vi "main.vi"() -> ()   [LabVIEW 2012]
panel:
  out "update flag":dbl[](array[numeric])
  out "Current Chart":dbl(graph)
  out "Temperature Chart":dbl(graph)
  in  "stop":bool
  in  "Pulse Width":dbl
  in  "Interlock":bool
  in  "Override":bool
  out "Laser Current":dbl(slide) scale=800.0..1024.0
  out "Laser Temperature":dbl(slide) scale=10.0..50.0
  in  "COMPort":refnum<visa-resource-name>
  in  "Input Source":bool
  in  "Period":dbl
  in  "Delay":dbl
  # "Internal"
  # "External"
  # "Interlock"
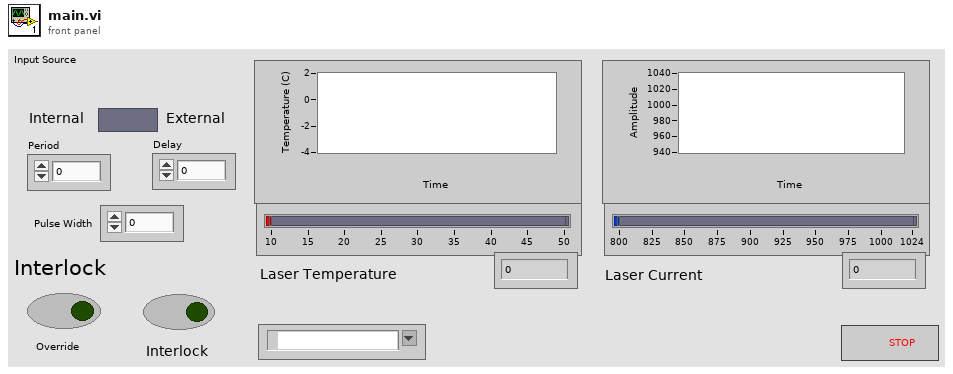
[diagram p1: front panel]
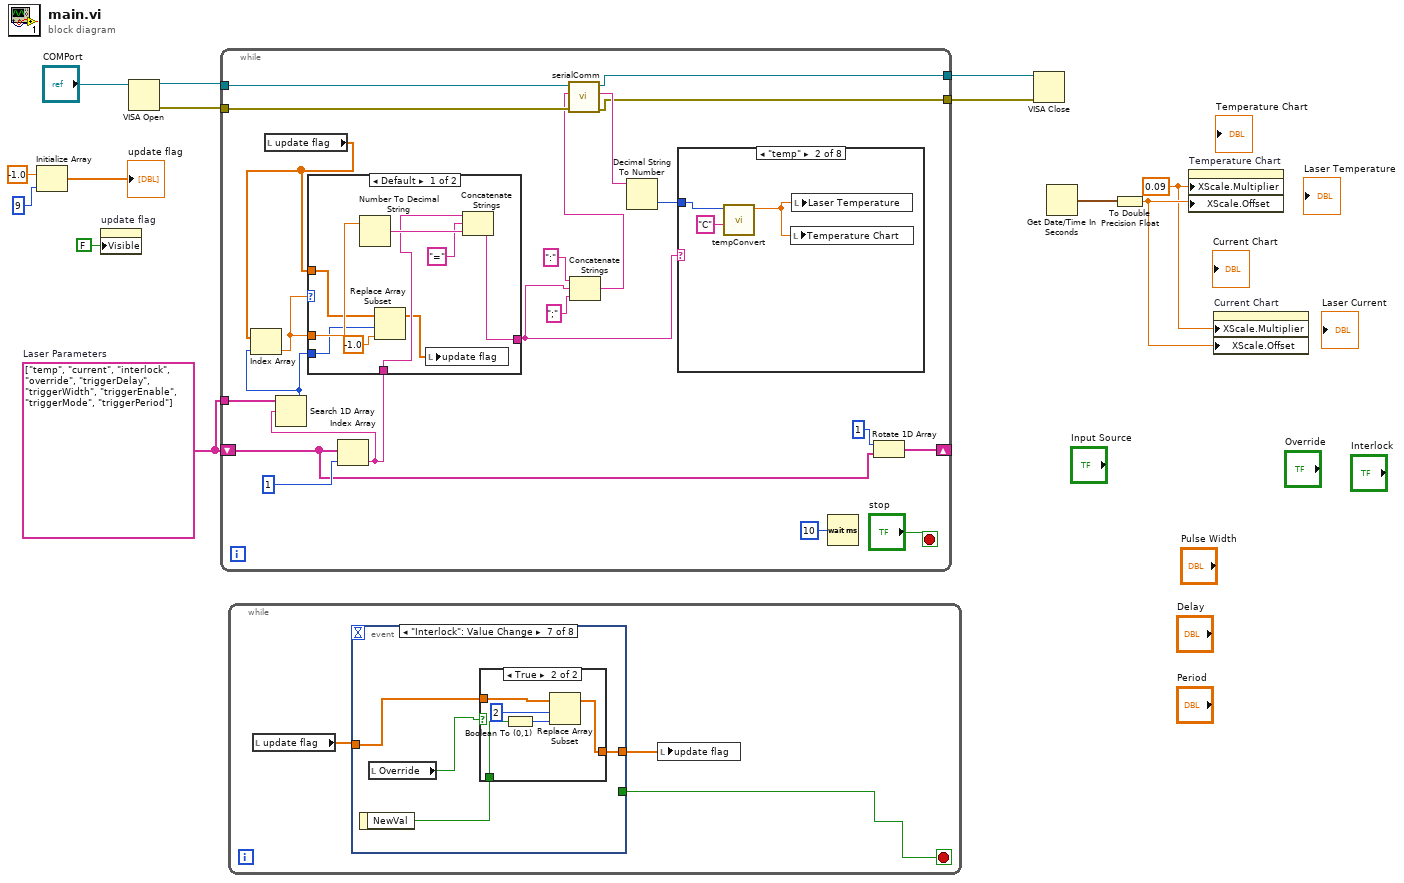
[diagram p0: block diagram]
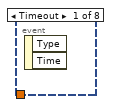
[diagram p2: hidden frame]
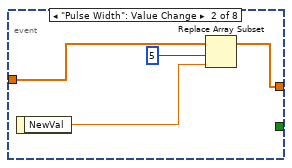
[diagram p3: hidden frame]
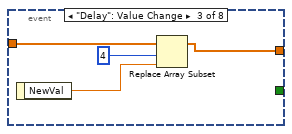
[diagram p4: hidden frame]
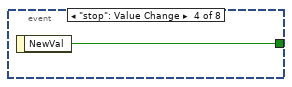
[diagram p5: hidden frame]
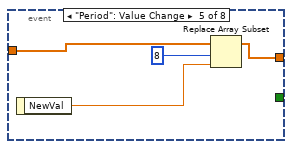
[diagram p6: hidden frame]
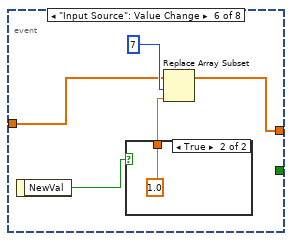
[diagram p7: hidden frame]
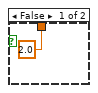
[diagram p8: hidden frame]
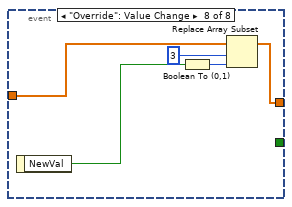
[diagram p10: hidden frame]
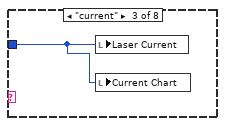
[diagram p13: hidden frame]
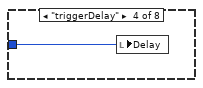
[diagram p14: hidden frame]
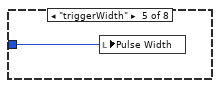
[diagram p15: hidden frame]
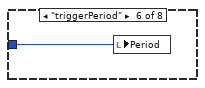
[diagram p16: hidden frame]
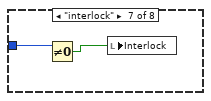
[diagram p17: hidden frame]
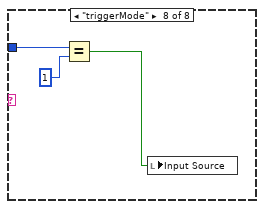
[diagram p18: hidden frame]
diagram:
  w6 = 0.09 ("X Scale.Offset and Multiplier:Multiplier")
  w5 = string[] ["temp", "current", "interlock", "override", "triggerDelay", "triggerWidth", "triggerEnable", "triggerMode", "triggerPeriod"]  # Laser Parameters
  n1 = Initialize Array(-1.0 ("element"), 9 ("dimension size")) -> (→"update flag":dbl[])
  n2 = property on="update flag" class="Arr (strict)"("Visible"=FALSE) -> ()  [unwired: 2 in, 2 out]
  n3 = VISA Open(VISA resource name="COMPort") -> (VISA resource name=w12:refnum<visa-resource-name>, error out=w11:errorcluster)  [unwired: 4 in]
  n4 = while {
    tunnel: w12 -> [w34]
    tunnel: w11 -> [w33]
    tunnel: [w30] -> w10
    tunnel: [w29] -> w9
    shift-right: [w15] -> _
    shift-left: w5 -> [w14]
    tunnel: w5 -> [w21]
    stop <- "stop" stop-if-true
    n5 = local read "update flag"() -> (w17:dbl[])
    n6 = Index Array(array=w14, index=1) -> (element=w20:string)
    n7 = Search 1D Array(1D array=w21, element=w20) -> (index of element=w16:i32)  [unwired: 1 in]
    n8 = Index Array(array=w17, index=w16) -> (element=w18:dbl)
    n9 = case shown="Default" w18 {
      tunnel: w20 -> [w38 w44]
      tunnel: [w43 w44] -> w19
      tunnel: w18 -> [w40 _]
      tunnel: w17 -> [w39 _]
      tunnel: w16 -> [w35 _]
      frame Default {
        n10 = Number To Decimal String(number=w40) -> (decimal integer string=w42:string)  [unwired: 1 in]
        n11 = Replace Array Subset(array=w39, new element=-1.0 ("new element/subarray"), index=w35) -> (w37:dbl[])
        n12 = local write "update flag"(w37) -> ()
        n13 = Concatenate Strings(w38, "=" ("string"), w42) -> (w43:string)
      }
      frame -1 {
      }
    }
    n14 = Concatenate Strings(":" ("string"), w19, ";" ("string")) -> (w22:string)
    n15 = call "serialComm.vi"("error in (no error)"=w33, "write buffer"=w22, "VISA resource name"=w34) -> ("error out"=w29:errorcluster, "read buffer"=w32:string, "VISA resource name 2"=w30:refnum<visa-resource-name>)  [unwired: 6 in]
    n16 = Decimal String To Number(string=w32) -> (number=w31:i32)  [unwired: 2 in, 1 out]
    n17 = case shown="\"temp\"" w19 {
      tunnel: w31 -> [_ w46 w48 w49 w50 w51 w53 w56]
      frame "False", Default {
      }
      frame "temp" {
        n18 = call "tempConvert.vi"("Units"="C", "ticks"=w46) -> ("value"=w47:dbl)  [unwired: 9 in]
        n19 = local write "Temperature Chart"(w47) -> ()
        n20 = local write "Laser Temperature"(w47) -> ()
      }
      frame "current" {
        n21 = local write "Laser Current"(w48) -> ()
        n22 = local write "Current Chart"(w48) -> ()
      }
      frame "triggerDelay" {
        n23 = local write "Delay"(w49) -> ()
      }
      frame "triggerWidth" {
        n24 = local write "Pulse Width"(w50) -> ()
      }
      frame "triggerPeriod" {
        n25 = local write "Period"(w51) -> ()
      }
      frame "interlock" {
        n26 = Not Equal To 0?(x=w53) -> (x != 0?=w52:bool)
        n27 = local write "Interlock"(w52) -> ()
      }
      frame "triggerMode" {
        n28 = Equal?(x=w56, y=1) -> (x = y?=w54:bool)
        n29 = local write "Input Source"(w54) -> ()
      }
    }
    n30 = Wait (ms)(milliseconds to wait=u32 10) -> ()  [unwired: 1 out]
    n31 = Rotate 1D Array(1:w14, 2:1 ("n")) -> (0:w15:string[])
  }
  n32 = while {
    stop <- w57 stop-if-true
    n33 = local read "update flag"() -> (w59:dbl[])
    n34 = event shown="[6] \"Interlock\": Value Change" {
      selector: _ -> [_ _ _ _ _ _ _ _]
      dyn-events: _ -> [_ _ _ _ _ _ _ _]
      timeout: _ -> [_ _ _ _ _ _ _ _]
      tunnel: w59 -> [_ w61 w67 _ w71 w74 w82 w93]
      tunnel: [_ w60 w65 _ w69 w75 w83 w92] -> w58
      tunnel: [_ _ _ w68 _ _ _ _] -> w57
      event Timeout {
        n35 = event-data() -> ()  [unwired: 1 in, 2 out]
      }
      event "Pulse Width": Value Change {
        n36 = event-data() -> ("NewVal"=w62:dbl)  [unwired: 1 in]
        n37 = Replace Array Subset(array=w61, new element=w62, index=5) -> (w60:dbl[])
      }
      event "Delay": Value Change {
        n38 = event-data() -> ("NewVal"=w64:dbl)  [unwired: 1 in]
        n39 = Replace Array Subset(array=w67, new element=w64, index=4) -> (w65:dbl[])
      }
      event "stop": Value Change {
        n40 = event-data() -> ("NewVal"=w68:bool)  [unwired: 1 in]
      }
      event "Period": Value Change {
        n41 = event-data() -> ("NewVal"=w70:dbl)  [unwired: 1 in]
        n42 = Replace Array Subset(array=w71, new element=w70, index=8) -> (w69:dbl[])
      }
      event "Input Source": Value Change {
        n43 = event-data() -> ("NewVal"=w77:bool)  [unwired: 1 in]
        n44 = case shown="True" w77 {
          tunnel: [2.0 ("new element/subarray") 1.0 ("new element/subarray")] -> w73
          frame False {
          }
          frame True {
          }
        }
        n45 = Replace Array Subset(array=w74, new element=w73, index=7) -> (w75:dbl[])
      }
      event "Interlock": Value Change {
        n46 = event-data() -> ("NewVal"=w81:bool)  [unwired: 1 in]
        n47 = local read "Override"() -> (w80:bool)
        n48 = case shown="True" w80 {
          tunnel: [w84 w87] -> w83
          tunnel: w82 -> [w84 w86]
          tunnel: w81 -> [_ w85]
          frame False {
          }
          frame True {
            n49 = Boolean To (0,1)(Boolean=w85) -> (0, 1=w88:i16)
            n50 = Replace Array Subset(array=w86, new element=w88, index=2) -> (w87:dbl[])
          }
        }
      }
      event "Override": Value Change {
        n51 = event-data() -> ("NewVal"=w90:bool)  [unwired: 1 in]
        n52 = Boolean To (0,1)(Boolean=w90) -> (0, 1=w91:i16)
        n53 = Replace Array Subset(array=w93, new element=w91, index=3) -> (w92:dbl[])
      }
    }
    n54 = local write "update flag"(w58) -> ()
  }
  n55 = VISA Close(VISA resource name=w10, error in (no error)=w9) -> ()  [unwired: 1 out]
  n56 = Get Date/Time In Seconds() -> (seconds since 1Jan1904=w8:timestamp)
  n57 = To Double Precision Float(number=w8) -> (double precision float=w7:dbl)
  n58 = property on="Temperature Chart" class="WFChart (strict)"("XScale.Multiplier"=w6, "XScale.Offset"=w7) -> ()  [unwired: 2 in, 2 out]
  n59 = property on="Current Chart" class="WFChart (strict)"("XScale.Multiplier"=w6, "XScale.Offset"=w7) -> ()  [unwired: 2 in, 2 out]
